vi "D_Window_Term.vi"(7 "Window Number (0...15)":i32, 8 "error in (no error)":errorcluster) -> (0 "error out":errorcluster)   [LabVIEW 2016]
uses:
  LabVIEW2018/Image_Control.dll
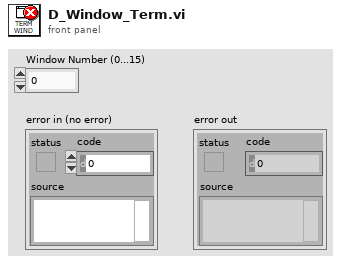
[diagram p1: front panel]
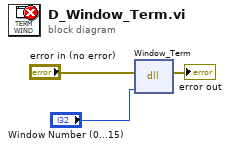
[diagram p0: block diagram]
diagram:
  n1 = dll-call lib="C:/Users/hs5921/Desktop/LabVIEW2018/Image_Control.dll" fn="Window_Term"(error in="error in (no error)", "WindowNum"="Window Number (0...15)") -> (error out=→"error out":errorcluster)  [unwired: 4 in, 1 out]
